vi "Globals.vi"() -> ()   [LabVIEW 2014]
panel:
  in  "Time 3":dbl
  in  "Time 2":dbl
  in  "FLAG":bool
  in  "Time":dbl
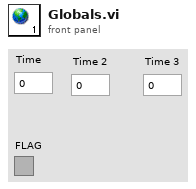
[diagram p1: front panel]
diagram:
